vi "Set LSS Pop Up.vi"(10 "Theme Choice":T1, 11 "Front Panel Objects":refnum<vi>[](array[refnum])) -> ()   [LabVIEW 2019, in "LSS.lvlib"]
doc: "Set style for front panel using LSS.\n\n<b>Inputs:</b>\n<b>Front Panel Objects</b> - Array of front panel controls that will have style applied to them.\n<b>Theme Choice</b> - Select theme that will be applied to front panel objects."
uses:
  LSS.lvlib
  Themes.ctl
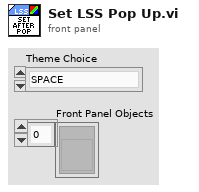
[diagram p1: front panel]
types:
  T1 = typedef "LSS.lvlib/Themes.ctl" = enum16{"SPACE", "ATK", "THEME1", "THEME2"}
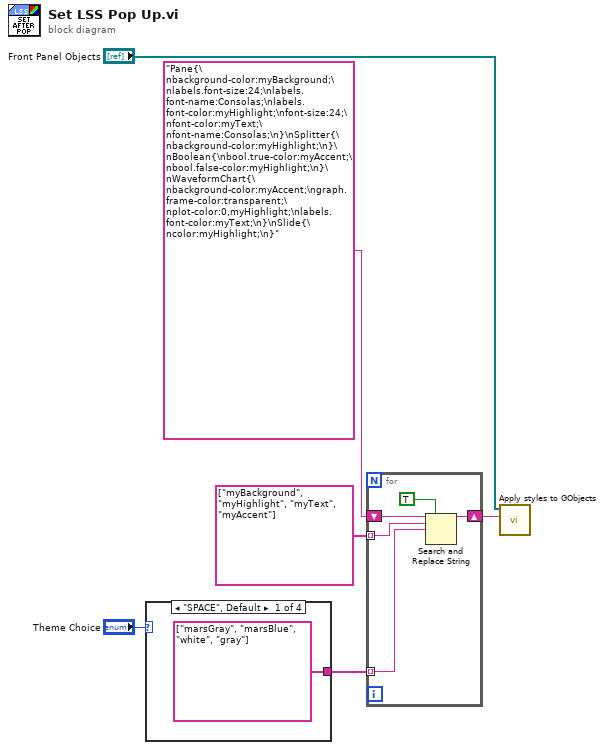
[diagram p0: block diagram]
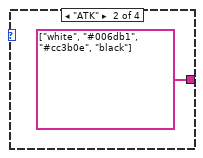
[diagram p2: hidden frame]
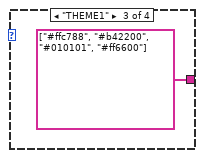
[diagram p3: hidden frame]
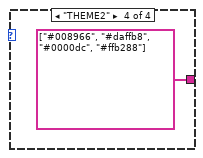
[diagram p4: hidden frame]
diagram:
  n1 = case shown="\"SPACE\", Default" "Theme Choice" {
    tunnel: [string[] ["marsGray", "marsBlue", "white", "gray"] string[] ["white", "#006db1", "#cc3b0e", "black"] string[] ["#ffc788", "#b42200", "#010101", "#ff6600"] string[] ["#008966", "#daffb8", "#0000dc", "#ffb288"]] -> w4
    frame "SPACE", Default {
    }
    frame "ATK" {
    }
    frame "THEME1" {
    }
    frame "THEME2" {
    }
  }
  n2 = for {
    tunnel: w4 -> [w11] mode=indexing
    tunnel: string[] ["myBackground", "myHighlight", "myText", "myAccent"] -> [w12] mode=indexing
    shift-right: [w13] -> w1
    shift-left: "Pane{\nbackground-color:myBackground;\nlabels.font-size:24;\nlabels.font-name:Consolas;\nlabels.font-color:myHighlight;\nfont-size:24;\nfont-color:myText;\nfont-name:Consolas;\n}\nSplitter{\nbackground-color:myHighlight;\n}\nBoolean{\nbool.true-color:myAccent;\nbool.false-color:myHighlight;\n}\nWaveformChart{\nbackground-color:myAccent;\ngraph.frame-color:transparent;\nplot-color:0,myHighlight;\nlabels.font-color:myText;\n}\nSlide{\ncolor:myHighlight;\n}" ("String") -> [w14]
    n3 = Search and Replace String(replace all?=TRUE ("replace all? (F)"), input string=w14, search string=w12, replace string=w11) -> (result string=w13:string)  [unwired: 4 in, 3 out]
  }
  n4 = call "Apply styles to GObjects.vi"("Style Sheet"=w1, "Front Panel Objects"="Front Panel Objects") -> ()  [unwired: 8 in, 2 out]
